vi "Identification.vi"(0 "MVEBRA":dbl, 5 "Data For Ident From OPC":dbl[][](array[numeric]), 7 "Prony\n approximation zone":enum16{"3/4 zone", "1/2 zone", "1/3 zone"}(ring), 9 "Select Method":enum16{"Transient Response", "Proni"}(ring)) -> (4 "Control object parameters  W(p) out":T2, 6 "Àverage error":dbl, 8 "Xoutput":dbl[](array[numeric]), 10 "Array":T1(array[cluster]))   [LabVIEW 2014]
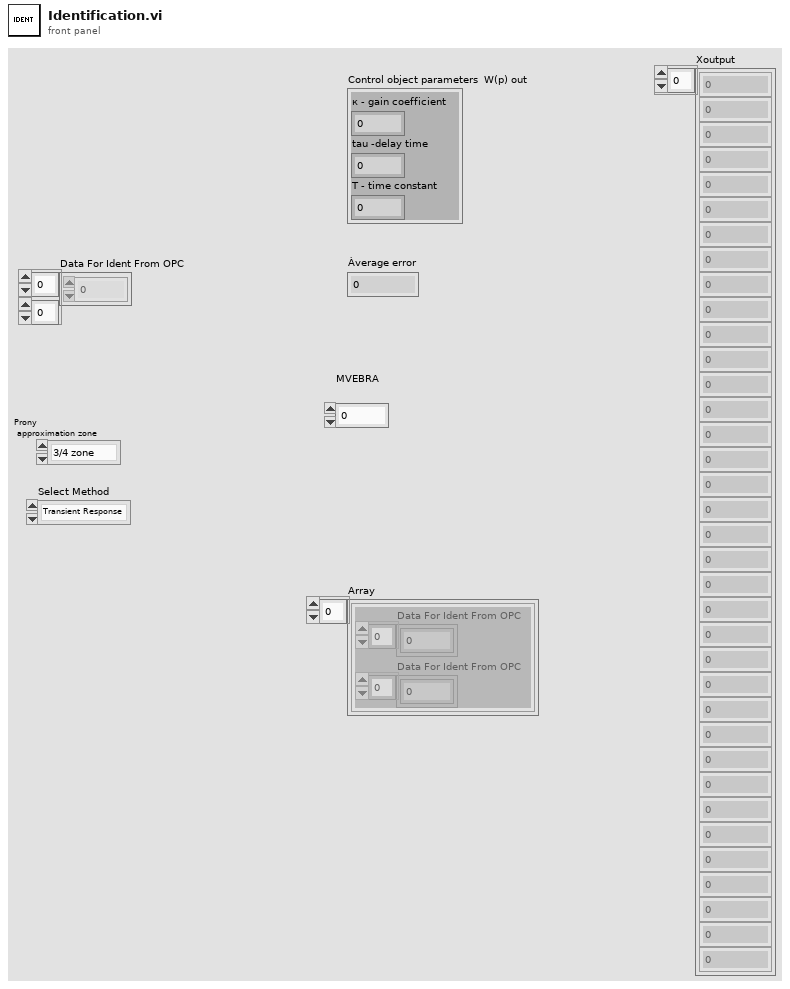
[diagram p1: front panel]
types:
  T1 = cluster{"Data For Ident From OPC":dbl[], "Data For Ident From OPC":dbl[]}[]
  T2 = cluster{"ê - gain coefficient":dbl, "tau -delay time":dbl, "T - time constant":dbl}
  T3 = cluster{"Data For Ident From OPC":dbl[], "Data For Ident From OPC":dbl[]}
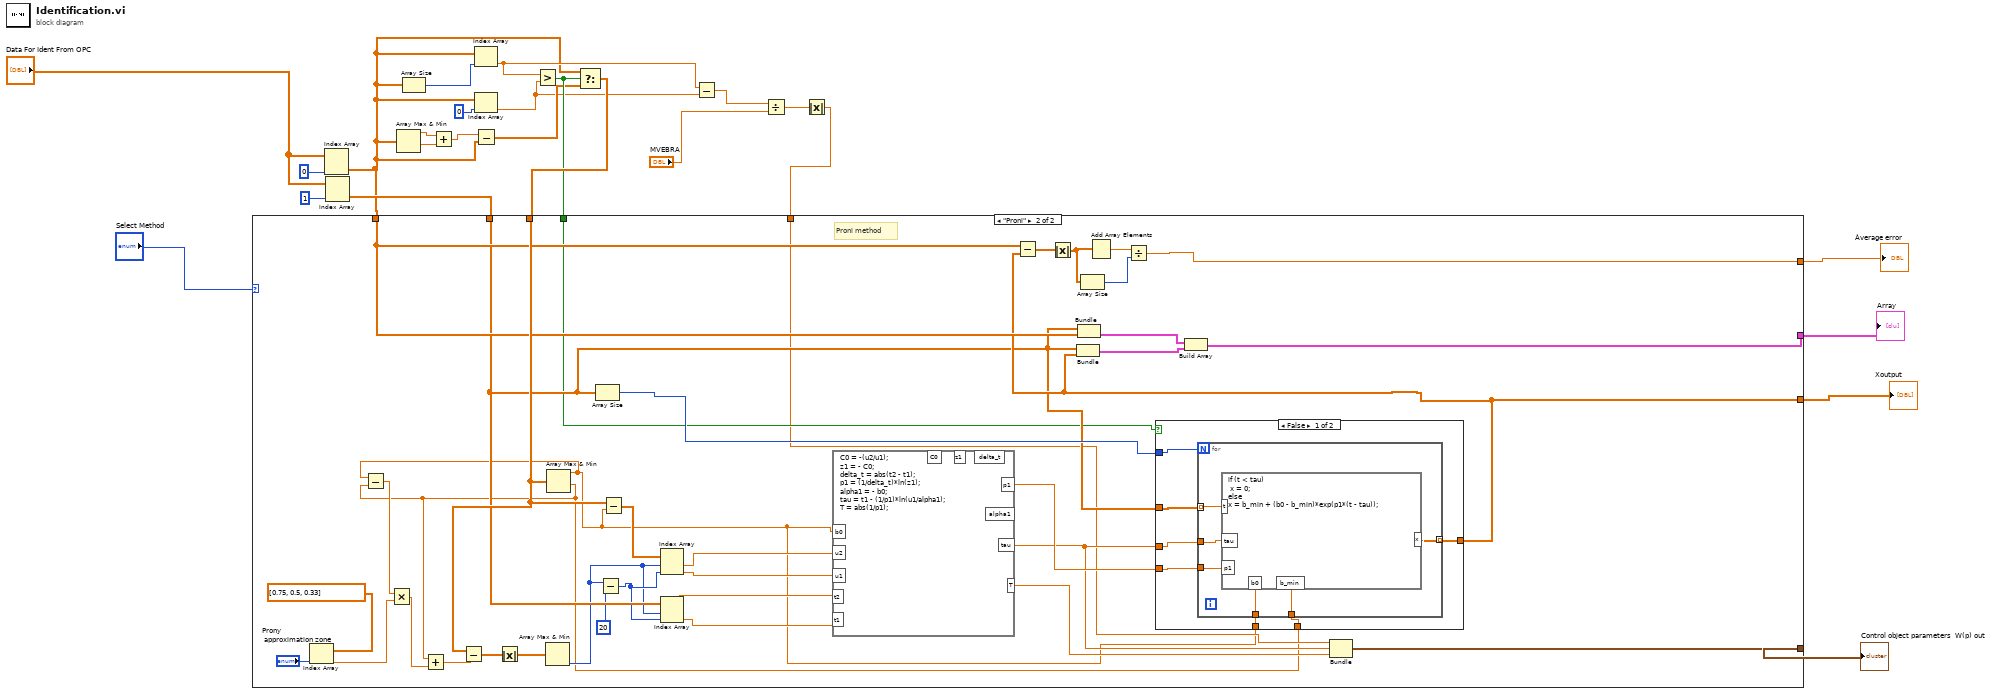
[diagram p0: block diagram]
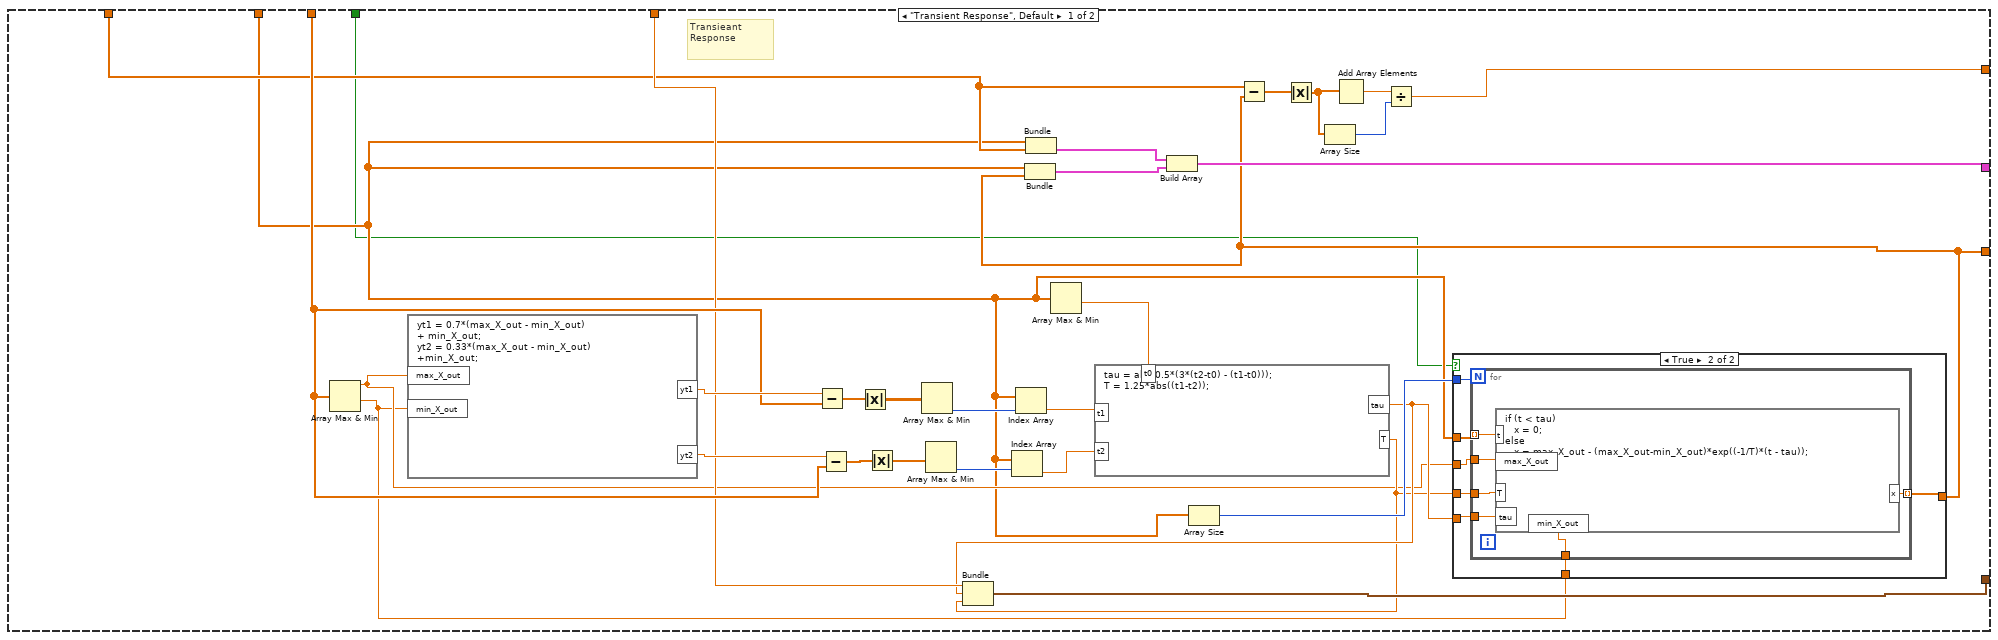
[diagram p2: hidden frame]
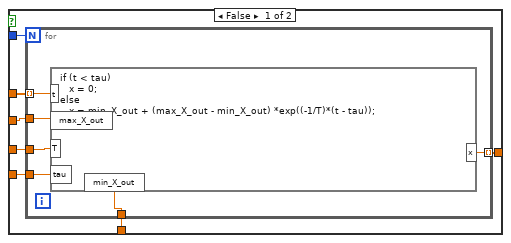
[diagram p3: hidden frame]
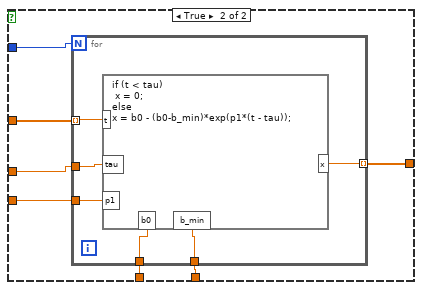
[diagram p4: hidden frame]
diagram:
  n1 = Index Array(array="Data For Ident From OPC", index (col)=0 ("disabled index (col)")) -> (element=w1:dbl[])  [unwired: 1 in]
  n2 = Index Array(array="Data For Ident From OPC", index (col)=1 ("disabled index (col)")) -> (element=w22:dbl[])  [unwired: 1 in]
  n3 = Array Max & Min(array=w1) -> (max value=w4:dbl, min value=w3:dbl)  [unwired: 2 out]
  n4 = Array Size(array=w1) -> (size(s)=w13:i32)
  n5 = Add(x=w4, y=w3) -> (x+y=w2:dbl)
  n6 = Index Array(array=w1, index=w13) -> (element=w9:dbl)
  n7 = Index Array(array=w1, index=0) -> (element=w8:dbl)
  n8 = Subtract(x=w2, y=w1) -> (x-y=w11:dbl[])
  n9 = Greater?(x=w9, y=w8) -> (0:w12:bool)
  n10 = Select(t=w1, s=w12, f=w11) -> (s? t:f=w14:dbl[])
  n11 = Subtract(x=w9, y=w8) -> (x-y=w10:dbl)
  n12 = Divide(x=w10, y="MVEBRA") -> (x/y=w7:dbl)
  n13 = Absolute Value(x=w7) -> (abs(x)=w5:dbl)
  n14 = case shown="\"Proni\"" "Select Method" {
    tunnel: [w53 w116] -> w18
    tunnel: w22 -> [w27 w94]
    tunnel: w14 -> [w40 w104]
    tunnel: [w35 w100] -> w23
    tunnel: [w36 w101] -> w17
    tunnel: [w28 w98] -> w16
    tunnel: w1 -> [w33 w99]
    tunnel: w12 -> [w26 w93]
    tunnel: w5 -> [w34 w92]
    frame "Transient Response", Default {
      # "Transieant Response"
      n15 = Array Max & Min(array=w40) -> (max value=w29:dbl, min value=w25:dbl)  [unwired: 2 out]
      n16 = formula code="yt1 = 0.7*(max_X_out - min_X_out) \n+ min_X_out;\nyt2 = 0.33*(max_X_out - min_X_out)\n+min_X_out;"("max_X_out"=w29, "min_X_out"=w25) -> ("yt1"=w42:dbl, "yt2"=w41:dbl)
      n17 = Subtract(x=w42, y=w40) -> (x-y=w48:dbl[])
      n18 = Subtract(x=w41, y=w40) -> (x-y=w47:dbl[])
      n19 = Absolute Value(x=w48) -> (abs(x)=w46:dbl[])
      n20 = Absolute Value(x=w47) -> (abs(x)=w43:dbl[])
      n21 = Array Max & Min(array=w46) -> (min index (indices)=w45:i32)  [unwired: 3 out]
      n22 = Array Max & Min(array=w43) -> (min index (indices)=w44:i32)  [unwired: 3 out]
      n23 = Index Array(array=w27, index=w44) -> (element=w39:dbl)
      n24 = Index Array(array=w27, index=w45) -> (element=w38:dbl)
      n25 = Bundle("Data For Ident From OPC"=w27, "Data For Ident From OPC"=w33) -> (w54:T3)  [unwired: 1 in]
      n26 = Array Max & Min(array=w27) -> (min value=w37:dbl)  [unwired: 3 out]
      n27 = formula code="tau = abs(0.5*(3*(t2-t0) - (t1-t0)));\nT = 1.25*abs((t1-t2));"("t1"=w38, "t2"=w39, "t0"=w37) -> ("tau"=w31:dbl, "T"=w30:dbl)
      n28 = Bundle(w34, "tau"=w31, "T"=w30) -> (w35:cluster{dbl, "tau":dbl, "T":dbl})  [unwired: 1 in]
      n29 = Array Size(array=w27) -> (size(s)=w32:i32)
      n30 = case shown="True" w26 {
        tunnel: w32 -> [w62 w75]
        tunnel: w31 -> [w61 w73]
        tunnel: w30 -> [w60 w72]
        tunnel: w29 -> [w59 w70]
        tunnel: [w58 w71] -> w28
        tunnel: w27 -> [w57 w74]
        tunnel: w25 -> [w56 w69]
        frame False {
          n31 = for {
            N: w62 -> [_]
            tunnel: w57 -> [w68] mode=indexing
            tunnel: w59 -> [w67]
            tunnel: [w66] -> w58 mode=indexing
            tunnel: w61 -> [w65]
            tunnel: w60 -> [w64]
            tunnel: w56 -> [w63]
            n32 = formula code="if (t < tau)\n   x = 0;\nelse\n   x = min_X_out + (max_X_out - min_X_out) *exp((-1/T)*(t - tau));"("tau"=w65, "max_X_out"=w67, "T"=w64, "t"=w68, "min_X_out"=w63) -> ("x"=w66:dbl)
          }
        }
        frame True {
          n33 = for {
            N: w75 -> [_]
            tunnel: w74 -> [w81] mode=indexing
            tunnel: w70 -> [w80]
            tunnel: [w79] -> w71 mode=indexing
            tunnel: w73 -> [w78]
            tunnel: w72 -> [w77]
            tunnel: w69 -> [w76]
            n34 = formula code="if (t < tau)\n   x = 0;\nelse\n   x = max_X_out - (max_X_out-min_X_out)*exp((-1/T)*(t - tau));"("tau"=w78, "max_X_out"=w80, "T"=w77, "t"=w81, "min_X_out"=w76) -> ("x"=w79:dbl)
          }
        }
      }
      n35 = Bundle("Data For Ident From OPC"=w27, w28) -> (w55:cluster{"Data For Ident From OPC":dbl[], dbl[]})  [unwired: 1 in]
      n36 = Build Array(w54, w55) -> (w53:T1)
      n37 = Subtract(x=w33, y=w28) -> (x-y=w49:dbl[])
      n38 = Absolute Value(x=w49) -> (abs(x)=w50:dbl[])
      n39 = Array Size(array=w50) -> (size(s)=w51:i32)
      n40 = Add Array Elements(numeric array=w50) -> (sum=w52:dbl)
      n41 = Divide(x=w52, y=w51) -> (x/y=w36:dbl)
    }
    frame "Proni" {
      # "Proni method"
      n42 = Index Array(array=dbl[] [0.75, 0.5, 0.33], index="Prony\n approximation zone") -> (element=w84:dbl)
      n43 = Array Max & Min(array=w104) -> (max value=w87:dbl, min value=w82:dbl)  [unwired: 2 out]
      n44 = Subtract(x=w87, y=w82) -> (x-y=w85:dbl)
      n45 = Multiply(x=w85, y=w84) -> (x*y=w83:dbl)
      n46 = Add(x=w82, y=w83) -> (x+y=w86:dbl)
      n47 = Subtract(x=w104, y=w86) -> (x-y=w106:dbl[])
      n48 = Absolute Value(x=w106) -> (abs(x)=w105:dbl[])
      n49 = Array Max & Min(array=w105) -> (min index (indices)=w90:i32)  [unwired: 3 out]
      n50 = Array Size(array=w94) -> (size(s)=w95:i32)
      n51 = Subtract(x=w90, y=20) -> (x-y=w91:i32)
      n52 = Subtract(x=w104, y=w87) -> (x-y=w115:dbl[])
      n53 = Index Array(array=w115, index #1=w90, index #2=w91) -> (element #1=w88:dbl, element #2=w113:dbl)
      n54 = Index Array(array=w94, index #1=w90, index #2=w91) -> (element #1=w114:dbl, element #2=w112:dbl)
      n55 = formula code="C0 = -(u2/u1);\nz1 = - C0;\ndelta_t = abs(t2 - t1);\np1 = (1/delta_t)*ln(z1);\nalpha1 = - b0;\ntau = t1 - (1/p1)*ln(u1/alpha1);\nT = abs(1/p1);"("u2"=w88, "u1"=w113, "b0"=w87, "t2"=w114, "t1"=w112) -> ("p1"=w97:dbl, "tau"=w96:dbl, "T"=w107:dbl)  [unwired: 4 out]
      n56 = Bundle("Data For Ident From OPC"=w94, "Data For Ident From OPC"=w99) -> (w118:T3)  [unwired: 1 in]
      n57 = case shown="False" w93 {
        tunnel: [w121 w138] -> w98
        tunnel: w97 -> [w122 w137]
        tunnel: w96 -> [w123 w136]
        tunnel: w95 -> [w125 w135]
        tunnel: w94 -> [w124 w134]
        tunnel: w87 -> [w120 w133]
        tunnel: w82 -> [w119 w132]
        frame False {
          n58 = for {
            N: w125 -> [_]
            tunnel: w123 -> [w131]
            tunnel: w124 -> [w130] mode=indexing
            tunnel: [w129] -> w121 mode=indexing
            tunnel: w122 -> [w128]
            tunnel: w120 -> [w127]
            tunnel: w119 -> [w126]
            n59 = formula code="if (t < tau)\n x = 0;\nelse\nx = b_min + (b0 - b_min)*exp(p1*(t - tau));"("tau"=w131, "t"=w130, "b0"=w127, "p1"=w128, "b_min"=w126) -> ("x"=w129:dbl)
          }
        }
        frame True {
          n60 = for {
            N: w135 -> [_]
            tunnel: w136 -> [w144]
            tunnel: w134 -> [w143] mode=indexing
            tunnel: [w142] -> w138 mode=indexing
            tunnel: w137 -> [w141]
            tunnel: w133 -> [w140]
            tunnel: w132 -> [w139]
            n61 = formula code="if (t < tau)\n x = 0;\nelse\nx = b0 - (b0-b_min)*exp(p1*(t - tau));"("tau"=w144, "t"=w143, "b0"=w140, "p1"=w141, "b_min"=w139) -> ("x"=w142:dbl)
          }
        }
      }
      n62 = Subtract(x=w99, y=w98) -> (x-y=w108:dbl[])
      n63 = Absolute Value(x=w108) -> (abs(x)=w109:dbl[])
      n64 = Bundle("Data For Ident From OPC"=w94, w98) -> (w117:cluster{"Data For Ident From OPC":dbl[], dbl[]})  [unwired: 1 in]
      n65 = Array Size(array=w109) -> (size(s)=w110:i32)
      n66 = Add Array Elements(numeric array=w109) -> (sum=w111:dbl)
      n67 = Divide(x=w111, y=w110) -> (x/y=w101:dbl)
      n68 = Build Array(w118, w117) -> (w116:T1)
      n69 = Bundle(w92, "tau"=w96, "T"=w107) -> (w100:cluster{dbl, "tau":dbl, "T":dbl})  [unwired: 1 in]
    }
  }
  "Control object parameters  W(p) out" <- w23
  "Array" <- w18
  "Àverage error" <- w17
  "Xoutput" <- w16
